vi "RIO_FinishUp.vi"(2 "Stack in":string[](array[string]), 3 "Stack in":string[](array[string])) -> (0 "Stack out":string[](array[string]), 1 "Stack out":string[](array[string]))   [LabVIEW 2012]
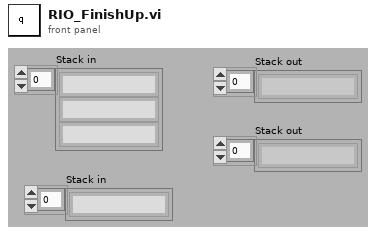
[diagram p1: front panel]
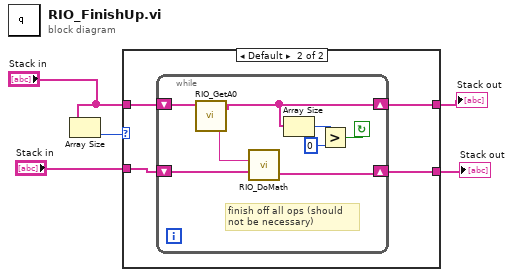
[diagram p0: block diagram]
diagram:
  n1 = Array Size(array="Stack in") -> (size(s)=w1:i32)
  n2 = case shown="Default" w1 {
    tunnel: [w7 w11] -> w5
    tunnel: "Stack in" -> [w6 w10]
    tunnel: [w6 w9] -> w3
    tunnel: "Stack in" -> [w7 w8]
    frame 0 {
    }
    frame Default {
      n3 = while {
        shift-right: [w19] -> w9
        shift-left: w10 -> [w18]
        shift-right: [w16] -> w11
        shift-left: w8 -> [w17]
        stop <- w12 continue-if-true
        # "finish off all ops (should\nnot be necessary)"
        n4 = call <userlib>:"RIO_GetA0.vi"("A[0..n]"=w17) -> ("A[1..n]"=w16:string[], "A[0]"=w15:string)
        n5 = call <userlib>:"RIO_DoMath.vi"("Stack in"=w18, "Last Operation"=w15) -> ("Stack out"=w19:string[])  [unwired: 1 in, 1 out]
        n6 = Array Size(array=w16) -> (size(s)=w14:i32)
        n7 = Greater?(x=w14, y=0) -> (0:w12:bool)
      }
    }
  }
  "Stack out" <- w5
  "Stack out" <- w3
